vi "initialize.vi"(2 "error in (no error)":errorcluster, 3 "VISA resource name in":refnum<visa-resource-name>="GPIB0::14::INSTR") -> (0 "error out":errorcluster, 1 "VISA Resource Name out":refnum<visa-resource-name>="GPIB0::14::INSTR")   [LabVIEW 2019]
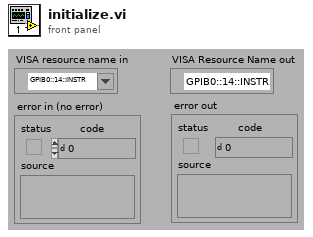
[diagram p1: front panel]
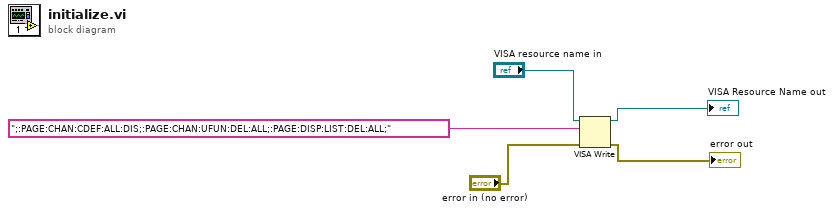
[diagram p0: block diagram]
diagram:
  n1 = VISA Write(VISA resource name="VISA resource name in", write buffer=";:PAGE:CHAN:CDEF:ALL:DIS;:PAGE:CHAN:UFUN:DEL:ALL;:PAGE:DISP:LIST:DEL:ALL;", error in (no error)="error in (no error)") -> (VISA resource name out=→"VISA Resource Name out":refnum<visa-resource-name>, error out=→"error out":errorcluster)  [unwired: 1 out]
